vi "Initialize References.vi"(8 "Description":refnum<vi>, 9 "Version":refnum<vi>, 10 "Status":refnum<vi>, 11 "Calling VI":refnum<vi>) -> (3 "Calling VI References":T1)   [LabVIEW 2021, in "TemplateCoreUtilities.lvlib"]
uses:
  TemplateCoreUtilities.lvlib
  Typedef/Calling VI References.ctl
  <vilib>/CIF Foundation/CIF LabVIEW Scripting/LV Scripting/Typedef/Version.ctl
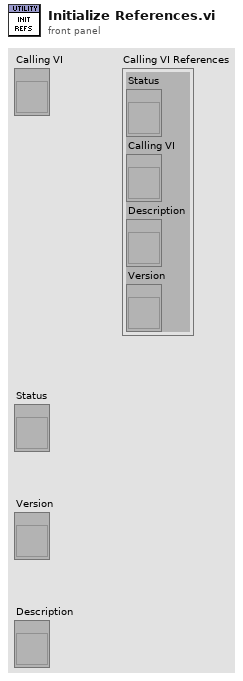
[diagram p1: front panel]
types:
  T1 = typedef "TemplateCoreUtilities.lvlib/Calling VI References.ctl" = cluster{"Status":refnum<vi>, "Calling VI":refnum<vi>, "Description":refnum<vi>, "Version":refnum<vi>}
  T2 = typedef "Version.ctl" = cluster{"Major":u16, "Minor":u16, "Fix":u16, "Build":u16}
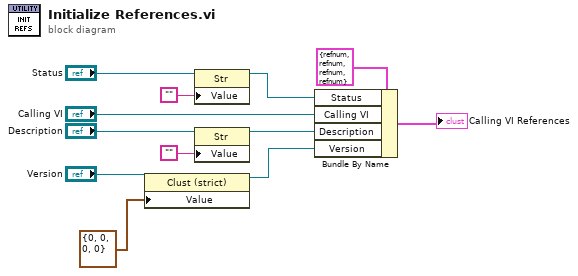
[diagram p0: block diagram]
diagram:
  n1 = property class="Clust (strict)"(reference="Version", "Value"=T2 {"Major"=0, "Minor"=0, "Fix"=0, "Build"=0}) -> (reference out=w1:refnum<vi>)  [unwired: 1 in, 1 out]
  n2 = property class="Str"(reference="Status", "Value"="") -> (reference out=w7:refnum<vi>)  [unwired: 1 in, 1 out]
  n3 = property class="Str"(reference="Description", "Value"="") -> (reference out=w4:refnum<vi>)  [unwired: 1 in, 1 out]
  n4 = Bundle By Name(cluster=T1 {"Status"=refnum, "Calling VI"=refnum, "Description"=refnum, "Version"=refnum} ("Calling VI References"), "Status"=w7, "Calling VI"="Calling VI", "Description"=w4, "Version"=w1) -> (→"Calling VI References":T1)
